vi "VIS-IR_ReadringBlock.vi"(6 "pixel":u32=1, 8 "error in (no error)":errorcluster, 9 "stop":i32, 10 "start":i32=1, 11 "VIS-IR in":refnum<class "VIS-NIR.lvclass">) -> (0 "error out":errorcluster, 2 "Data Values":u32[][](graph), 3 "VIS-IR out":refnum<class "VIS-NIR.lvclass">)   [LabVIEW 2015, in "VIS-NIR.lvclass"]
uses:
  VIS-NIR.lvclass
  Detector.lvclass/Detector.ctl
  Detector.lvclass
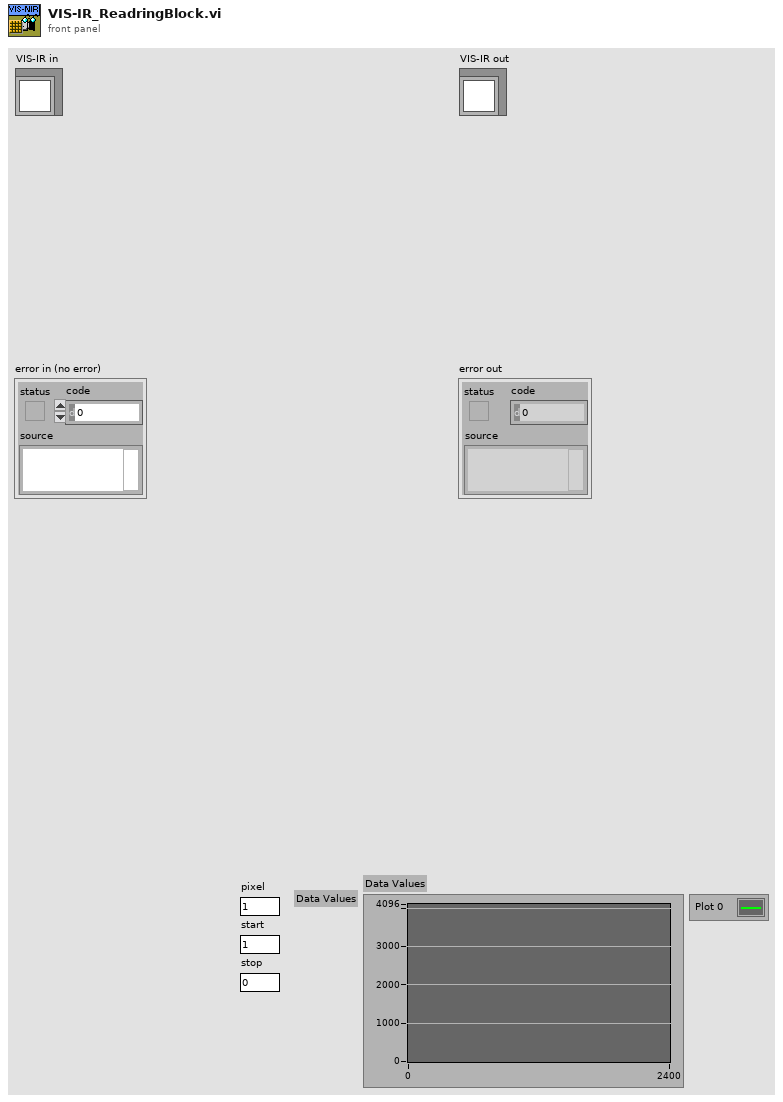
[diagram p1: front panel]
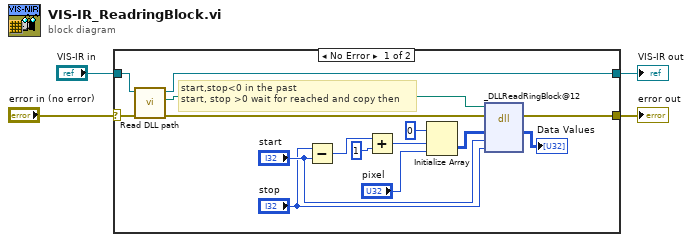
[diagram p0: block diagram]
diagram:
  n1 = case shown="No Error" "error in (no error)" {
    selector: "error in (no error)" -> [w18 w21]
    tunnel: [w10 w21] -> w3
    tunnel: [w6 w20] -> w1
    tunnel: "VIS-IR in" -> [w19 w20]
    frame No Error {
      # "start,stop<0 in the past\nstart, stop >0 wait for reached and copy then"
      n2 = call "Read DLL path.vi"("error in (no error)"=w18, "Detector in"=w19) -> ("error out"=w11:errorcluster, "DLL path"=w5:path, "Detector out"=w6:refnum<class "VIS-NIR.lvclass">)  [unwired: 7 in]
      n3 = Subtract(x="stop", y="start") -> (x-y=w15:i32)
      n4 = Add(x=w15, y=1) -> (x+y=w14:i32)
      n5 = Initialize Array(u32 0, w14, "pixel") -> (w7:u32[][])
      n6 = dll-call lib="G:/SD/TRANCON/DLL/ESLSCDLL.dll" fn="_DLLReadRingBlock@12" ("lwlscdll.dll:DLLReadLoop")(path in=w5, error in=w11, "dioden"=w7, "start"="start", "stop"="stop") -> (error out=w10:errorcluster, "dioden"=→"Data Values":u32[][])  [unwired: 4 in, 1 out]
    }
    frame Error {
    }
  }
  "error out" <- w3
  "VIS-IR out" <- w1
